vi "Mcp2210 Set Manufacturer String.vi"(8 "error in (no error)":errorcluster, 10 "Manufacturer":string, 11 "handle":i32) -> (0 "error out":errorcluster, 3 "handle out":i32)   [LabVIEW 2015, in "mcp2210.lvlib"]
doc: "Write the USB Manufacturer string into device NVRAM.\nIn case of successful execution, the function returns 0 (M_E_SUCCESS).\nIn case of failure, negative error code is returned.\nIf the error code is \"M_E_ERR_BLOCKED_ACCESS\" the write failure is due to the device being either\npassword protected or permanently locked. M_Mcp2210_GetAccessStatus() API provides the details about\ndevice protection status. If the device is not permanently locked, the password protection can be\nunlocked or disabled by using the access control API.\nParameters:\nInputs:\n- IntPtr handle - USB device handle. Cannot be NULL.\n- String ^manufacturerStr - String object containing the manufacturer UNICODE string.\nCannot be NULL.\n!! Important detail !!\n- maximum string length must be 29 UNICODE characters without\ncounting the NULL termination (M_MCP2210_DESCRIPTOR_STR_MAX_LEN).\nIf the input string is larger, negative error code is returned.\nOutputs:\n- none\nReturns:\n- 0 for success: M_E_SUCCESS\n- negative error code: M_E_ERR_NULL, M_E_ERR_INVALID_HANDLE_VALUE\nM_E_ERR_STRING_TOO_LARGE\nM_E_ERR_HID_TIMEOUT, M_E_ERR_HID_RW_FILEIO, M_E_ERR_UNKOWN_ERROR\nM_E_ERR_CMD_ECHO, M_E_ERR_CMD_FAILED\nM_E_ERR_BLOCKED_ACCESS\n\nMCP2210_DLL_UM_API int __stdcall Mcp2210_SetManufacturerString(void *handle, unsigned short *manufacturerStr);"
uses:
  <userlib>/mcp2210/mcp2210.lvlib
  <userlib>/mcp2210/mcp2210_dll_um_x86.dll
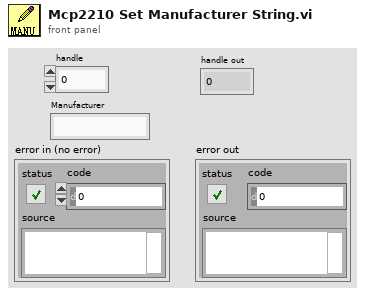
[diagram p1: front panel]
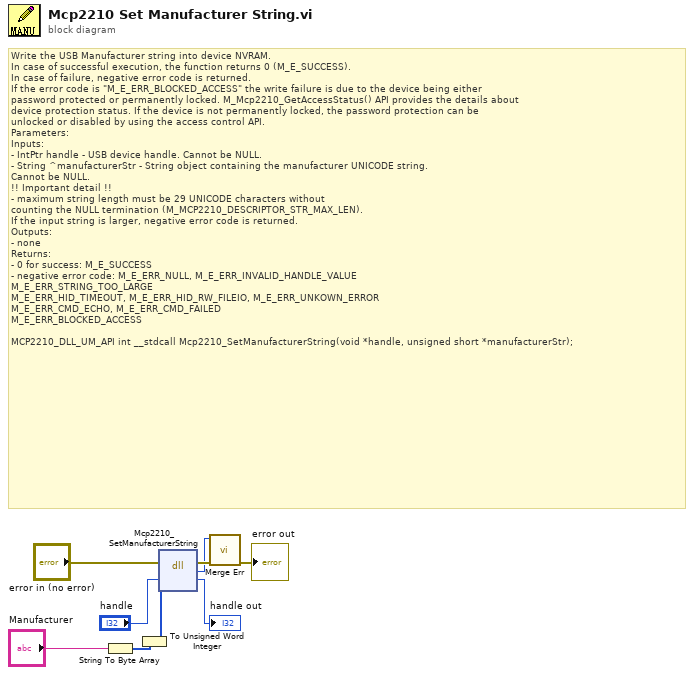
[diagram p0: block diagram]
diagram:
  # "Write the USB Manufacturer string into device NVRAM.\nIn case of successful execution, the function returns 0 (M_E_SUCCESS).\nIn case of failure, negative error code is returned.\nIf the error code is \"M_E_ERR_BLOCKED_ACCESS\" the write failure is due to the device being either\npassword protected or permanently locked. M_Mcp2210_GetAccessStatus() API provides the details about\ndevice protection status. If the device is not permanently locked, the password protection can be\nunlocked or disabled by using the access control API.\nParameters:\nInputs:\n- IntPtr handle - USB device handle. Cannot be NULL.\n- String ^manufacturerStr - String object containing the manufacturer UNICODE string.\nCannot be NULL.\n!! Important detail !!\n- maximum string length must be 29 UNICODE characters without\ncounting the NULL termination (M_MCP2210_DESCRIPTOR_STR_MAX_LEN).\nIf the input string is larger, negative error code is returned.\nOutputs:\n- none\nReturns:\n- 0 for success: M_E_SUCCESS\n- negative error code: M_E_ERR_NULL, M_E_ERR_INVALID_HANDLE_VALUE\nM_E_ERR_STRING_TOO_LARGE\nM_E_ERR_HID_TIMEOUT, M_E_ERR_HID_RW_FILEIO, M_E_ERR_UNKOWN_ERROR\nM_E_ERR_CMD_ECHO, M_E_ERR_CMD_FAILED\nM_E_ERR_BLOCKED_ACCESS\n\nMCP2210_DLL_UM_API int __stdcall Mcp2210_SetManufacturerString(void *handle, unsigned short *manufacturerStr);"
  n1 = String To Byte Array(string="Manufacturer") -> (unsigned byte array=w2:u8[])
  n2 = To Unsigned Word Integer(number=w2) -> (unsigned 16bit integer=w1:u16[])
  n3 = dll-call lib="D:/LabVIEW 2015/user.lib/mcp2210/mcp2210_dll_um_x86.*" fn="Mcp2210_SetManufacturerString"(error in="error in (no error)", "handle"="handle", "manufacturerStr"=w1) -> (error out=w7:errorcluster, "return type"=w6:i32, "handle"=→"handle out":i32)  [unwired: 3 in, 1 out]
  n4 = call <userlib>:"Merge Err.vi"("error in (no error)"=w7, "return type"=w6) -> ("error out"=→"error out":errorcluster)  [unwired: 9 in]
